vi "Load Animated GIF Image (Memory).vi"(8 "error in (no error)":errorcluster, 9 "Transparency Threshold (127)":u8=127, 11 "Encoded Image":u8[](array[numeric])) -> (0 "error out":errorcluster, 1 "Delays":i32[](array[numeric]), 2 "Frames":T1[](array[typedef]))   [LabVIEW 2020, in "G-Image.lvlib"]
doc: "Decodes the byte array to a LabVIEW picture."
uses:
  G-Image.lvlib
  <vilib>/picture/picture.llb/imagedata.ctl
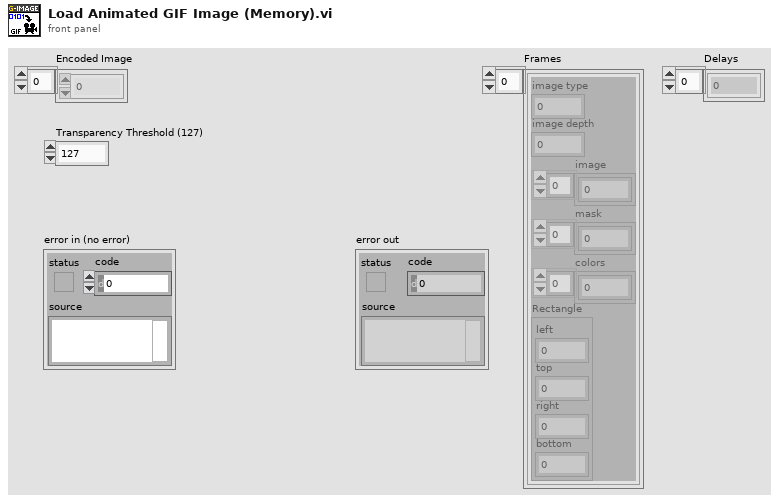
[diagram p1: front panel]
types:
  T1 = typedef "imagedata.ctl" = cluster{"image type":i32, "image depth":i32, "image":u8[], "mask":u8[], "colors":u32[], "Rectangle":cluster{"left":i16, "top":i16, "right":i16, "bottom":i16}}
  T2 = typedef "G-Image.lvlib/Extended Image.ctl" = cluster{"Image":T1, "Layers":i32, "Delays":i32[]}
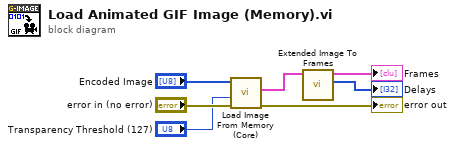
[diagram p0: block diagram]
diagram:
  n1 = call "Load Image From Memory (Core).vi"("error in (no error)"="error in (no error)", "Transparency Threshold (127)"="Transparency Threshold (127)", "Encoded Image"="Encoded Image") -> ("error out"=→"error out":errorcluster, "Extended Image"=w1:T2)  [unwired: 7 in]
  n2 = call "Extended Image To Frames.vi"("Extended Image"=w1) -> ("Delays"=→"Delays":i32[], "Frames"=→"Frames":T1[])  [unwired: 9 in]
